vi "Glimpse Generate Test Sequence.vi"() -> ()   [LabVIEW 2016]
uses:
  Sequence files handle.ctt
  Header2 file data.ctl
  Seq file v 1/Offset table.ctl
  Seq file v 1/Offset.ctl
  Seq file v 1/file number.ctl
  GLIMPSE Globals.vi
  <vilib>/vision/NI_Vision_Development_Module.lvlib
panel:
  in  "Number of acquisition files":i32=10
  in  "Number of frames to make":i32=20
  in  "Go? (F)":bool
  in  "New":bool
  in  "Over-write":bool=TRUE
  in  "Over-write exisitng:":path=path "d:/1.glimpse"
  in  "Digitize to new directory":path=path "d:/1.glimpse"
  in  "stop":bool
  out "Frames created":u32(slide) scale=0.0..20.0
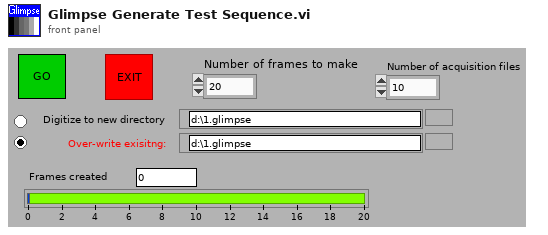
[diagram p1: front panel]
types:
  T1 = enum32{"8 bits", "16 bits", "Float", "Complex", "RGB Chunky", "Compressed"}
  T2 = typedef "Sequence files handle.ctt" = cluster{"Sequence files directory path":path, "Sequence files refnum array":refnum<file>[]}
  T3 = typedef "Offset table.ctl" = cluster{"offset":T4, "file number":T5}[]
  T4 = typedef "Offset.ctl" = i32
  T5 = typedef "file number.ctl" = u8
  T6 = enum32{"Frame", "Paint", "Invert Frame", "Invert Paint"}
  T7 = cluster{"desired font(Application)":enum16{"User-specified Font", "Application Font", "System Font", "Dialog Font"}, "[user-specified font]":cluster{"Font Name:":string, "Size":i16, "Strikeout?":bool, "Italic?":bool, "Underline?":bool, "Outline?":bool, "Shadow?":bool, "Bold?":bool}, "Alignment":i32}
  T8 = typedef "Header2 file data.ctl" = cluster{"Camera":string, "Microscope":string, "Microscope software version":string, "Laser names":string[], "Filter names":string[], "Lasers array":u16[][], "Filter array":u16[], "Flow rate array":dbl[], "Temperature array":dbl[], "Field array":u16[], "Is header2 info present?":bool, "Description Info":string, "Stage xyz array":dbl[][]}
  T9 = typedef "IMAQ Image.ctl" = refnum<image>
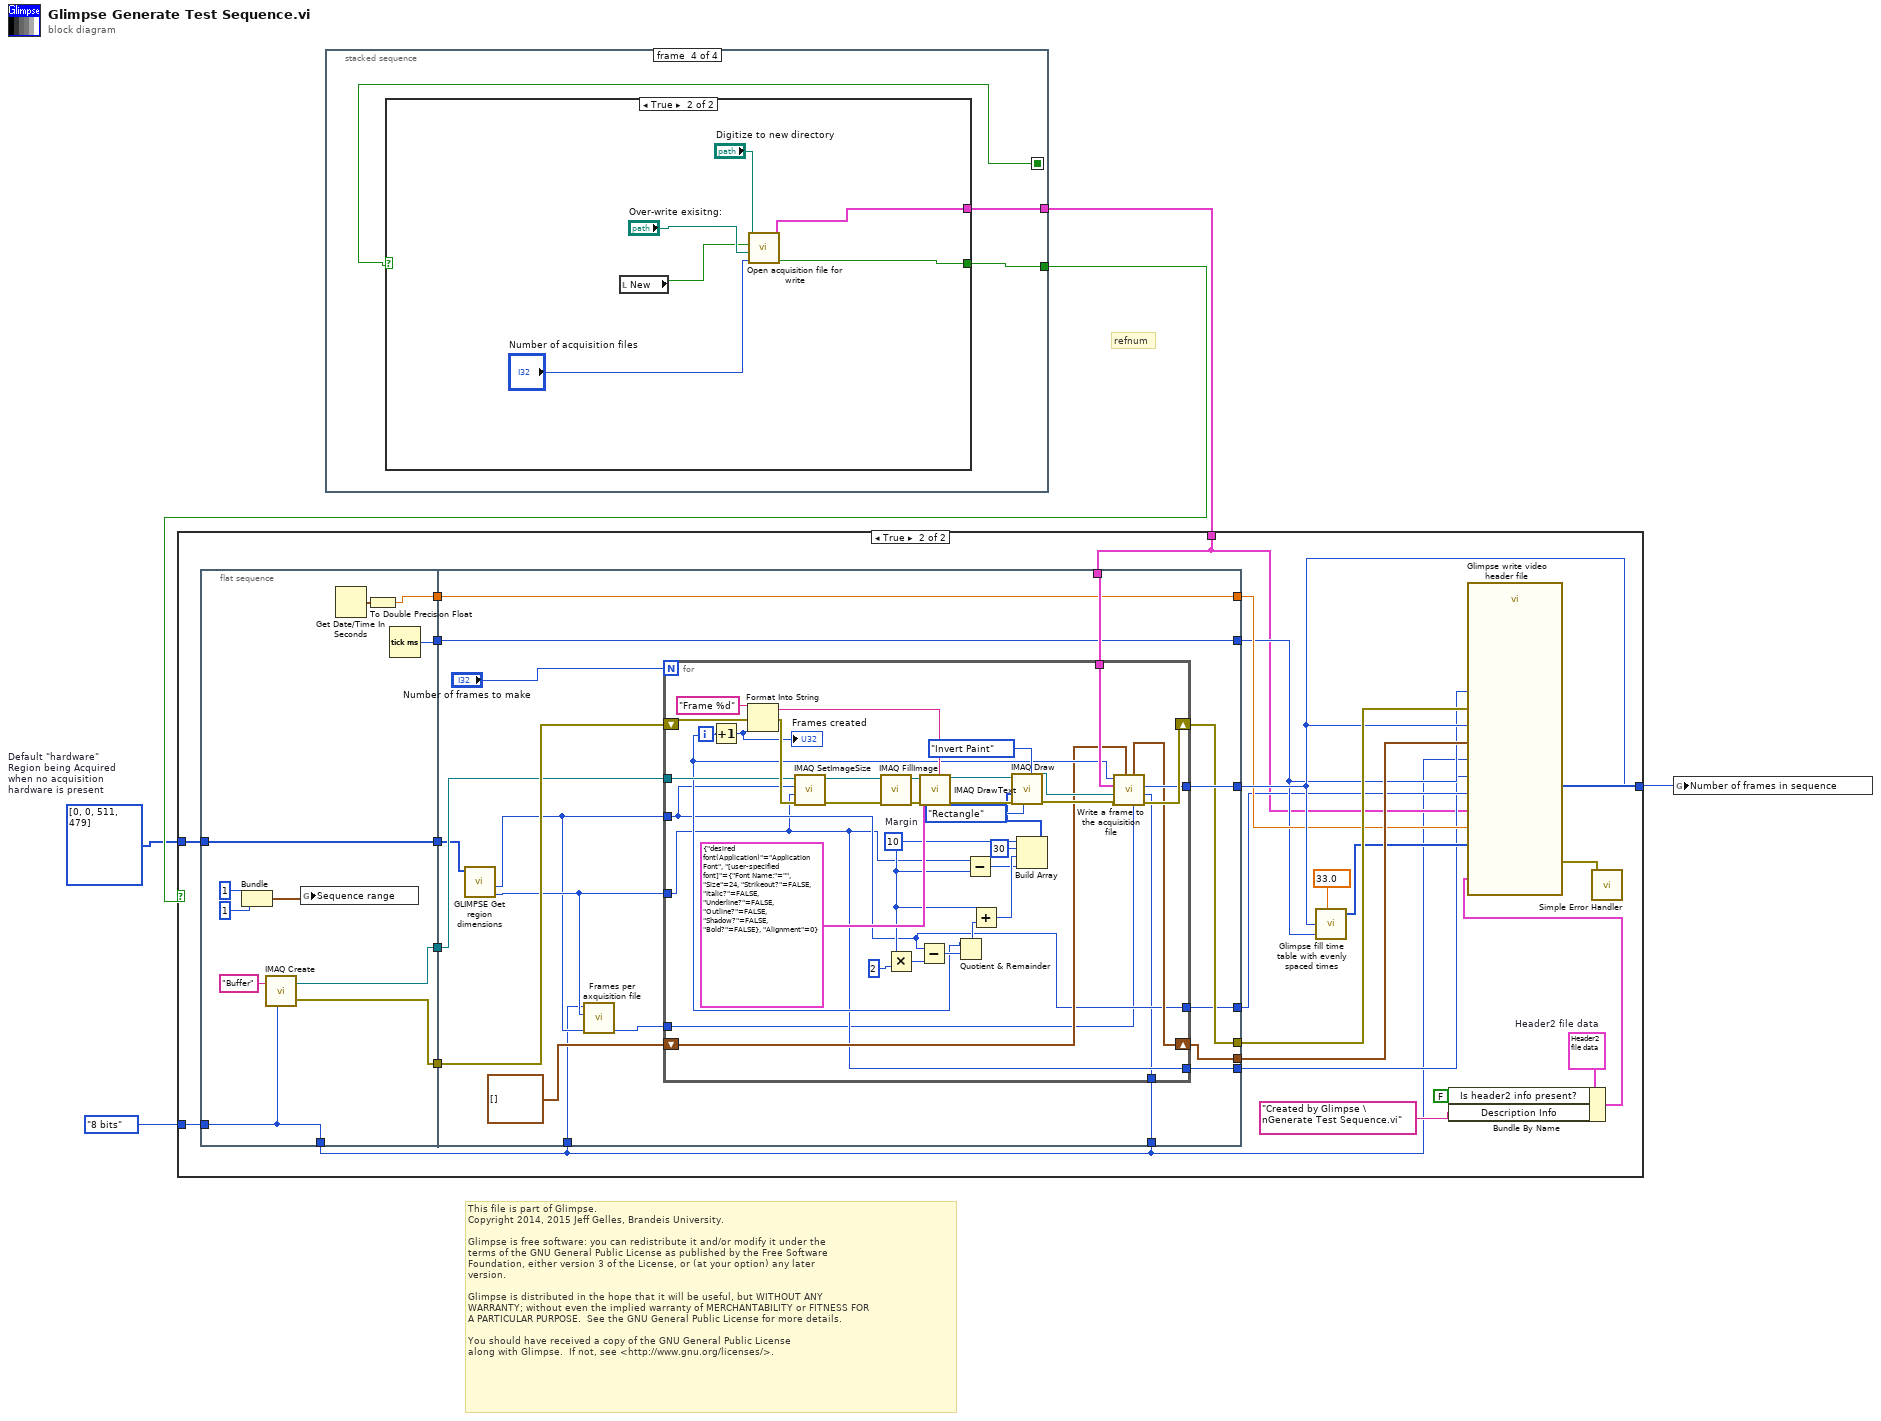
[diagram p0: block diagram]
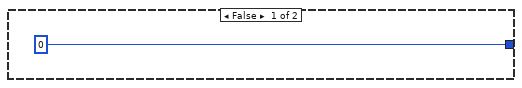
[diagram p2: hidden frame]
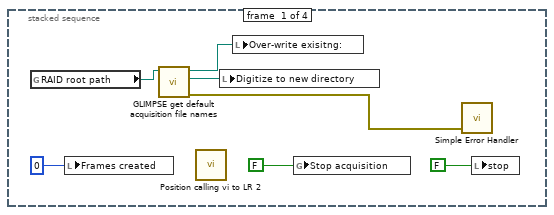
[diagram p3: hidden frame]
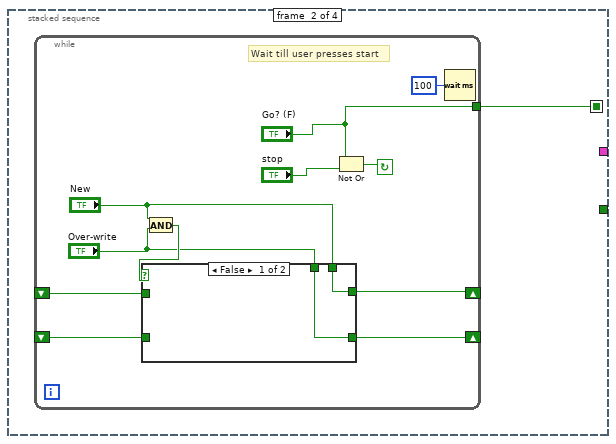
[diagram p4: hidden frame]
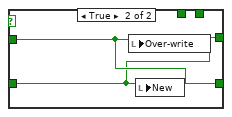
[diagram p5: hidden frame]
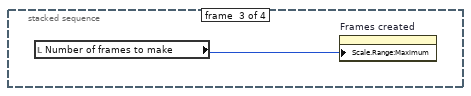
[diagram p6: hidden frame]
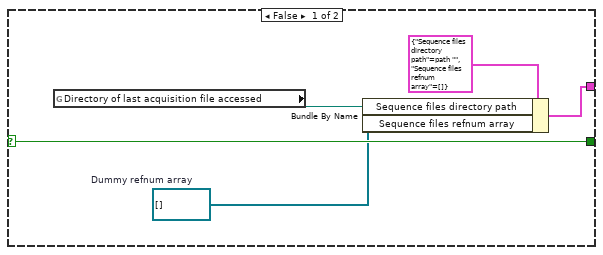
[diagram p7: hidden frame]
diagram:
  w2 = i32[] [0, 0, 511, 479]  # Default "hardware" Region being Acquired when no acquisition hardware is present
  # "This file is part of Glimpse. \nCopyright 2014, 2015 Jeff Gelles, Brandeis University.    \n\nGlimpse is free software: you can redistribute it and/or modify it under the \nterms of the GNU General Public License as published by the Free Software \nFoundation, either version 3 of the License, or (at your option) any later \nversion.\n\nGlimpse is distributed in the hope that it will be useful, but WITHOUT ANY \nWARRANTY; without even the implied warranty of MERCHANTABILITY or FITNESS FOR \nA PARTICULAR PURPOSE.  See the GNU General Public License for more details.\n\nYou should have received a copy of the GNU General Public License\nalong with Glimpse.  If not, see <http://www.gnu.org/licenses/>."
  # "refnum"
  n1 = stacked-sequence {
    seq-local: [_ w13 _ _] -> [_ _ _ w32]
    tunnel: [_ _ _ w31] -> w5
    tunnel: [_ _ _ w30] -> w3
    frame #0 {
      n2 = global read "GLIMPSE Globals.vi" "RAID root path"() -> (w10:path)
      n3 = local write "Frames created"(u32 0 ("Frames Acquired")) -> ()
      n4 = call "GLIMPSE get default acquisition file names.vi"("RAID root path"=w10) -> ("error out"=w9:errorcluster, "next directory path"=w8:path, "last directory path"=w7:path)  [unwired: 1 in, 5 out]
      n5 = call "Position calling vi to LR 2.vi"() -> ()  [unwired: 2 in, 4 out]
      n6 = local write "Digitize to new directory"(w8) -> ()
      n7 = local write "Over-write exisitng:"(w7) -> ()
      n8 = global write "GLIMPSE Globals.vi" "Stop acquisition"(FALSE ("Stop acquisition")) -> ()
      n9 = call <vilib>:"Simple Error Handler.vi"("error in (no error)"=w9) -> ()  [unwired: 1 in, 8 out]
      n10 = local write "stop"(FALSE ("stop")) -> ()
    }
    frame #1 {
      n11 = while {
        tunnel: ["Go? (F)"] -> w13
        shift-right: [w20] -> _
        shift-left: _ -> [w17]
        shift-right: [w18] -> _
        shift-left: _ -> [w16]
        stop <- w24 continue-if-true
        # "Wait till user presses start"
        n12 = And(x="New", y="Over-write") -> (x .and. y?=w22:bool)
        n13 = case shown="False" w22 {
          tunnel: [w26 w27] -> w20
          tunnel: "New" -> [w26 _]
          tunnel: "Over-write" -> [w25 _]
          tunnel: [w25 w28] -> w18
          tunnel: w17 -> [_ w28]
          tunnel: w16 -> [_ w27]
          frame False {
          }
          frame True {
            n14 = local write "Over-write"(w28) -> ()
            n15 = local write "New"(w27) -> ()
          }
        }
        n16 = Not Or(1:"stop", 2:"Go? (F)") -> (0:w24:bool)
        n17 = Wait (ms)(milliseconds to wait=u32 100) -> ()  [unwired: 1 out]
      }
    }
    frame #2 {
      n18 = local read "Number of frames to make"() -> (w29:i32)
      n19 = property on="Frames created" class="Slide (strict)"("Scale.Range:Maximum"=w29) -> ()  [unwired: 2 in, 2 out]
    }
    frame #3 {
      n20 = case shown="True" w32 {
        selector: w32 -> [w37 _]
        tunnel: [w37 w43] -> w31
        tunnel: [w34 w39] -> w30
        frame False {
          w35 = refnum<file>[] []  # Dummy refnum array
          n21 = global read "GLIMPSE Globals.vi" "Directory of last acquisition file accessed"() -> (w36:path)
          n22 = Bundle By Name(cluster=T2 {"Sequence files directory path"=path "", "Sequence files refnum array"=[]} ("Sequence files handle"), "Sequence files directory path"=w36, "Sequence files refnum array"=w35) -> (w34:T2)
        }
        frame True {
          n23 = local read "New"() -> (w40:bool)
          n24 = call "Open acquisition file for write.vi"("Number of acquisition files"="Number of acquisition files", "Existing directory to over-write"="Over-write exisitng:", "Use new?"=w40, "New directory to create"="Digitize to new directory") -> ("OK?"=w43:bool, "Sequence files handle"=w39:T2)  [unwired: 5 out]
        }
      }
    }
  }
  n25 = case shown="True" w5 {
    tunnel: [u32 0 ("Last frame number written out") w62] -> w4
    tunnel: w3 -> [_ w50]
    tunnel: w2 -> [_ w64]
    tunnel: T1."8 bits" ("Image Type") -> [_ w55]
    frame False {
    }
    frame True {
      w49 = T8 {"Camera"="", "Microscope"="", "Microscope software version"="", "Laser names"=[], "Filter names"=[], "Lasers array"=[], "Filter array"=[], "Flow rate array"=[], "Temperature array"=[], "Field array"=[], "Is header2 info present?"=FALSE, "Description Info"="", "Stage xyz array"=[]}  # Header2 file data
      n26 = flat-sequence {
        tunnel: w64 -> [w69]
        tunnel: [w69] -> w60
        tunnel: [w78] -> w59
        tunnel: [w73] -> w58
        tunnel: [w72] -> w57
        tunnel: [w70] -> w56
        tunnel: w55 -> [w68]
        tunnel: [w68] -> w45
        tunnel: [w94] -> w62
        tunnel: [w92] -> w67
        tunnel: [w91] -> w65
        tunnel: w60 -> [w89]
        tunnel: w59 -> [w87]
        tunnel: w58 -> [w95]
        tunnel: w57 -> [w96]
        tunnel: w56 -> [w86]
        tunnel: w50 -> [w88]
        tunnel: [w87] -> w53
        tunnel: [w86] -> w54
        tunnel: [w85] -> w52
        tunnel: [w84] -> w51
        tunnel: w45 -> [w83]
        tunnel: w45 -> [w79]
        frame #0 {
          n27 = Bundle(i16 1, i16 1) -> (w77:cluster{i16, i16})  [unwired: 1 out]
          n28 = call "IMAQ Create"("Image Name"="Buffer", "Image Type"=w68) -> ("New Image"=w73:T9, "error out"=w72:errorcluster)  [unwired: 2 in, 1 out]
          n29 = global write "GLIMPSE Globals.vi" "Sequence range"(w77) -> ()
          n30 = Get Date/Time In Seconds() -> (seconds since 1Jan1904=w71:timestamp)
          n31 = To Double Precision Float(number=w71) -> (double precision float=w70:dbl)
          n32 = Tick Count (ms)() -> (millisecond timer value=w78:u32)
        }
        frame #1 {
          n33 = call "GLIMPSE Get region dimensions.vi"("x1y1x2y2"=w89) -> ("y size"=w82:u16, "x size"=w81:u16)  [unwired: 9 out]
          n34 = call "Frames per axquisition file.vi"("Output frame width"=w81, "Output frame height"=w82, "Pixel depth"=w79) -> ("Frames per acquisition file"=w80:i32)  [unwired: 3 in, 1 out]
          n35 = for {
            N: "Number of frames to make" -> [_]
            shift-right: [w107] -> w91
            shift-left: w96 -> [w131]
            tunnel: w81 -> [w100]
            tunnel: w82 -> [w99]
            tunnel: w95 -> [w109]
            tunnel: w88 -> [w105]
            tunnel: [w104] -> w94
            shift-right: [w101] -> w92
            shift-left: T3 [] ("Offset table in") -> [w102]
            tunnel: [w100] -> w85
            tunnel: [w99] -> w84
            tunnel: w83 -> [w98]
            tunnel: w80 -> [w97]
            i -> [w103]
            w112 = 10  # Margin
            n36 = Increment(x=w103) -> (x+1=w110:i32)
            "Frames created" <- w110
            n37 = Format Into String(format string="Frame %d", error in=w131, w110) -> (resulting string=w130:string, error out=w125:errorcluster)  [unwired: 1 in]
            n38 = call "IMAQ SetImageSize"("error in (no error)"=w125, "Y Resolution"=w99, "X Resolution"=w100, "Image"=w109) -> ("error out"=w127:errorcluster, "Image Out"=w126:T9)  [unwired: 1 out]
            n39 = call "IMAQ FillImage"("error in (no error)"=w127, "Image"=w126) -> ("error out"=w129:errorcluster, "Image Out"=w128:T9)  [unwired: 5 in, 3 out]
            n40 = Multiply(x=w112, y=2) -> (x*y=w116:i32)
            n41 = Subtract(x=w100, y=w116) -> (x-y=w115:i32)
            n42 = call "IMAQ DrawText"("String"=w130, "error in (no error)"=w129, "Font, Size & Style"=T7 {"desired font(Application)"=enum."Application Font", "[user-specified font]"={"Font Name:"="", "Size"=24, "Strikeout?"=FALSE, "Italic?"=FALSE, "Underline?"=FALSE, "Outline?"=FALSE, "Shadow?"=FALSE, "Bold?"=FALSE}, "Alignment"=0}, "Image Src"=w128) -> ("error out"=w123:errorcluster, "Image Dst Out"=w122:T9)  [unwired: 3 in, 3 out]
            n43 = Quotient & Remainder(x=w103, y=w115) -> (x-y*floor(x/y)=w114:i32)  [unwired: 1 out]
            n44 = Subtract(x=w99, y=w112) -> (x-y=w111:i32)
            n45 = Add(x=w112, y=w114) -> (x+y=w113:i32)
            n46 = Build Array(w112, 30 ("Margin"), w113, w111) -> (w119:i32[])
            n47 = call "IMAQ Draw"("Draw Mode"=T6."Invert Paint", "Shape to draw"=enum32{"Line", "Rectangle", "Oval"}."Rectangle", "error in (no error)"=w123, "Coordinates"=w119, "Image Src"=w122) -> ("error out"=w108:errorcluster, "Image Dst Out"=w106:T9)  [unwired: 2 in, 3 out]
            n48 = call "Write a frame to the acquisition file.vi"("Pixel depth"=w98, "Frames per acquisition file"=w97, "Offset table in"=w102, "error in"=w108, "Image In"=w106, "Sequence files handle"=w105, "Last frame number written in"=w103) -> ("error out"=w107:errorcluster, "Last frame number written out"=w104:u32, "Offset table out"=w101:T3)  [unwired: 2 out]
          }
        }
      }
      n49 = call "Glimpse fill time table with evenly spaced times.vi"("Element 0 of TTB"=w53, "Number of frames in sequence"=w62, "Milliseconds per frame"=33.0) -> ("TTB Array"=w61:u32[])  [unwired: 2 out]
      n50 = Bundle By Name(cluster=w49, "Is header2 info present?"=FALSE, "Description Info"="Created by Glimpse \nGenerate Test Sequence.vi") -> (w46:T8)
      n51 = call "Glimpse write video header file.vi"("Number of frames"=w62, "Sequence files handle"=w50, "Pixel depth\n(0=8 bit; 1= 16 bit)"=w45, "error in"=w65, "TTB Array"=w61, "Offsets Array"=w67, "Header2 file data"=w46, "Region width"=w52, "Region height"=w51, "Element 0 of TTB"=w53, "time of 1st frame, \nsec since 1/1/04"=w54) -> ("error out"=w66:errorcluster)  [unwired: 8 in]
      n52 = call <vilib>:"Simple Error Handler.vi"("error in (no error)"=w66) -> ()  [unwired: 1 in, 8 out]
    }
  }
  n53 = global write "GLIMPSE Globals.vi" "Number of frames in sequence"(w4) -> ()
